vi "Configure Messaging.vi"(8 "error in (no error)":errorcluster, 10 "Msg Configuration":T1={"sendEndEn"=TRUE, "suppEnEnRd"=FALSE, "termChar"=13, "EnTermChar"=TRUE}, 11 "Serial Session in":refnum<class "Serial Session.lvclass">) -> (0 "error out":errorcluster, 3 "Serial Session out":refnum<class "Serial Session.lvclass">)   [LabVIEW 2015, in "Serial Session.lvclass"]
uses:
  Serial Session.lvclass
  Typedefs/Msg Config.ctl
  Serial Session.lvclass/Serial Session.ctl
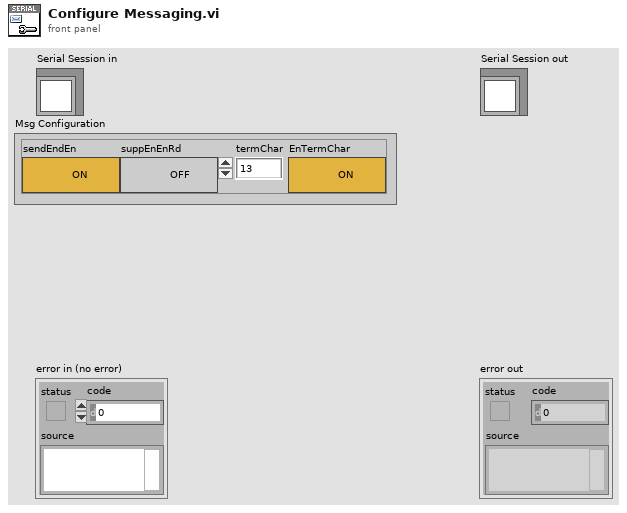
[diagram p1: front panel]
types:
  T1 = typedef "Serial Session.lvclass/Msg Config.ctl" = cluster{"sendEndEn":bool, "suppEnEnRd":bool, "termChar":u8, "EnTermChar":bool}
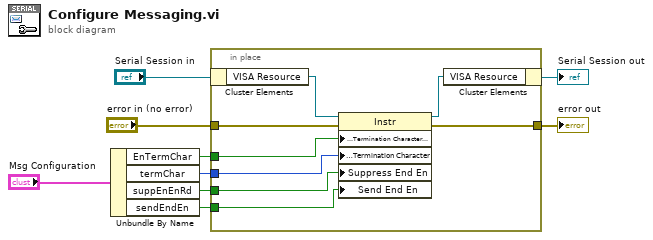
[diagram p0: block diagram]
diagram:
  n1 = Unbundle By Name("Msg Configuration") -> ("EnTermChar"=w9:bool, "termChar"=w8:u8, "suppEnEnRd"=w7:bool, "sendEndEn"=w6:bool)
  n2 = in-place {
    in-place-border: w9 -> [w17]
    in-place-border: w8 -> [w16]
    in-place-border: w7 -> [w15]
    in-place-border: w6 -> [w14]
    in-place-border: "error in (no error)" -> [w13]
    in-place-border: [w12] -> w4
    n3 = in-place-cluster #1("Serial Session in") -> ("VISA Resource"=w11:refnum<visa-resource-name>)
    n4 = property class="Instr"(reference=w11, error in=w13, "Message Based Settings:Termination Character Enable"=w17, "Message Based Settings:Termination Character"=w16, "Suppress End En"=w15, "Send End En"=w14) -> (reference out=w10:refnum<visa-resource-name>, error out=w12:errorcluster)
    n5 = in-place-cluster #1("VISA Resource"=w10) -> (→"Serial Session out":refnum<class "Serial Session.lvclass">)
  }
  "error out" <- w4
